vi "Read Magnetic Field.vi"(8 "error in (no error)":errorcluster, 11 "Honeywell Compass HMC6343":refnum<class "Honeywell Compass HMC6343.lvclass">) -> (0 "error out":errorcluster, 2 "Magnetic Field":T1, 3 "Honeywell Compass HMC6343 out":refnum<class "Honeywell Compass HMC6343.lvclass">)   [LabVIEW 2019, in "Honeywell Compass HMC6343.lvclass"]
doc: "Reads Magnetic Field."
uses:
  Honeywell Compass HMC6343.lvclass
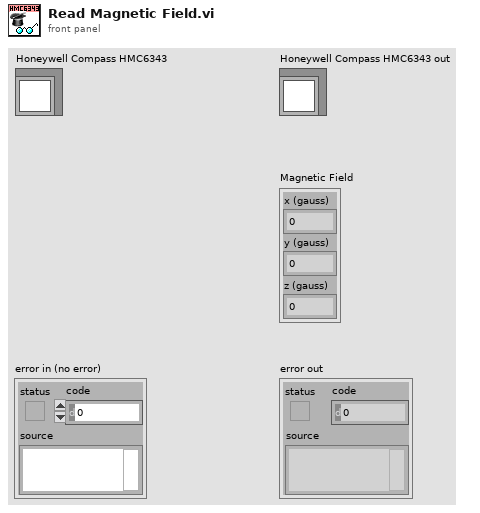
[diagram p1: front panel]
types:
  T1 = cluster{"x (gauss)":dbl, "y (gauss)":dbl, "z (gauss)":dbl}
  T2 = cluster{"Head (deg)":dbl, "Pitch (deg)":dbl, "Roll (deg)":dbl}
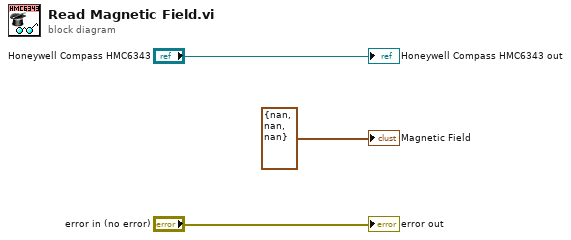
[diagram p0: block diagram]
diagram:
  "error out" <- "error in (no error)"
  "Honeywell Compass HMC6343 out" <- "Honeywell Compass HMC6343"
  "Magnetic Field" <- T2 {"Head (deg)"=nan, "Pitch (deg)"=nan, "Roll (deg)"=nan} ("Heading Data")
